vi "TestExec.Read Local Station, Get Xlink Options.vi"(8 "error in":errorcluster, 11 "Config File Path":path) -> (0 "error out":errorcluster, 3 "Overall Results Only":bool)   [LabVIEW 2018]
uses:
  <vilib>/Utility/config.llb/Read Key (Boolean).vi
  <vilib>/Utility/config.llb/NI_LVConfig.lvlib
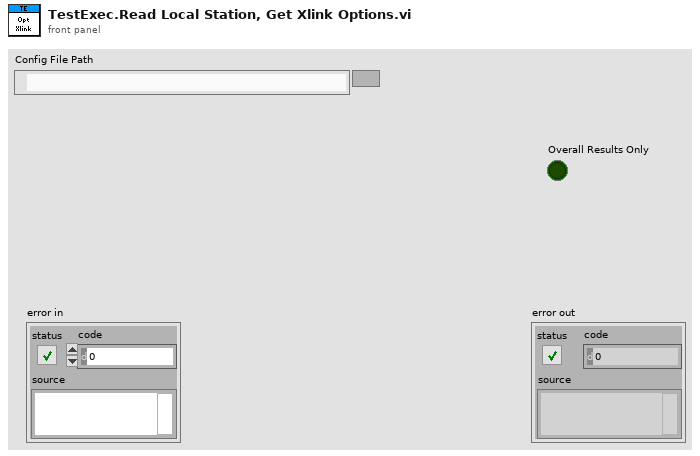
[diagram p1: front panel]
types:
  T1 = typedef "NI_LVConfig.lvlib/Config Data RefNum.ctl" = refnum<k1>
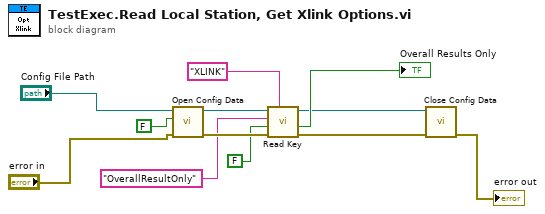
[diagram p0: block diagram]
diagram:
  n1 = call <vilib>:"Open Config Data.vi"("error in (no error)"="error in", "create file if necessary (T)"=FALSE, "configuration file path"="Config File Path") -> ("error out"=w10:errorcluster, "refnum"=w11:T1)  [unwired: 6 in, 1 out]
  n2 = call-poly <vilib>:"Read Key.vi"("section"="XLINK", "error in (no error)"=w10, "default value"=FALSE ("create file if necessary (T)"), "key"="OverallResultOnly", "refnum"=w11) -> ("error out"=w1:errorcluster, "value"=→"Overall Results Only":bool, "refnum out"=w2:T1)  [unwired: 3 in, 1 out]
  n3 = call <vilib>:"Close Config Data.vi"("error in (no error)"=w1, "refnum"=w2) -> ("error out"=→"error out":errorcluster)  [unwired: 8 in, 1 out]
